vi "Graph Average Temptature.vi"() -> ()   [LabVIEW 2015]
panel:
  in  "On/Off":bool=TRUE
  out "Waveform Chart":cluster{dbl, "Temperature":dbl}(graph)
  # "ON"
  # "OFF"
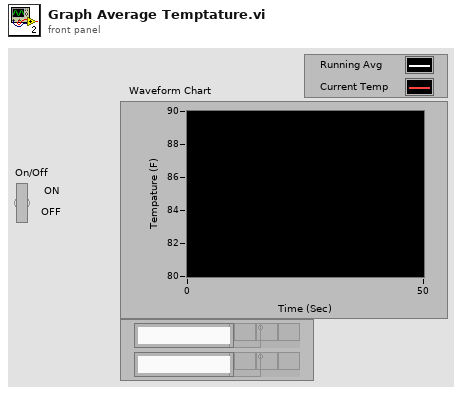
[diagram p1: front panel]
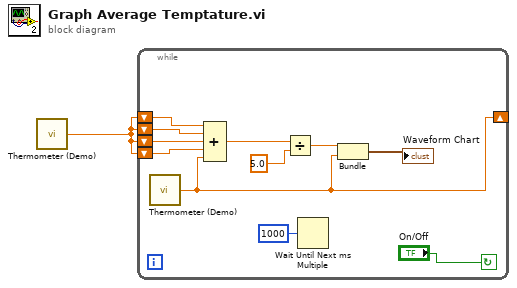
[diagram p0: block diagram]
diagram:
  n1 = call "Thermometer (Demo).vi"() -> ("Temperature"=w1:dbl)  [unwired: 1 in]
  n2 = while {
    shift-right: [w2] -> _
    shift-left: w1 -> [w11]
    shift-left: w1 -> [w10]
    shift-left: w1 -> [w9]
    shift-left: w1 -> [w8]
    stop <- "On/Off" continue-if-true
    n3 = call "Thermometer (Demo).vi"() -> ("Temperature"=w2:dbl)  [unwired: 1 in]
    n4 = Compound Arithmetic op=ADD(w11, w10, w9, w8, w2) -> (w6:dbl)
    n5 = Divide(x=w6, y=5.0) -> (x/y=w4:dbl)
    n6 = Wait Until Next ms Multiple(millisecond multiple=u32 1000) -> ()  [unwired: 1 out]
    n7 = Bundle(w4, "Temperature"=w2) -> (→"Waveform Chart":cluster{dbl, "Temperature":dbl})  [unwired: 1 in]
  }
